vi "FTW-Actor-Core-Initialize.vi"(0 "FTW Actor Instance":refnum<class "FTW-Actor-Instance.lvclass">, 5 "Inbox Configuration":string, 7 "Primary Inbox Address":string, 9 "Actor Identity":string, 11 "error in":errorcluster) -> (4 "FTW Actor Instance out":refnum<class "FTW-Actor-Instance.lvclass">, 6 "Incoming Request":refnum<event-registration>, 8 "Resolved Primary Inbox Address":string, 15 "error out":errorcluster)   [LabVIEW 2015, in "FTW-Actor-Instance.lvclass"]
uses:
  FTW-Actor-Instance.lvclass
  core/type/FTW-Type-JSON.ctl
panel:
  # "Inputs"
  # "Outputs"
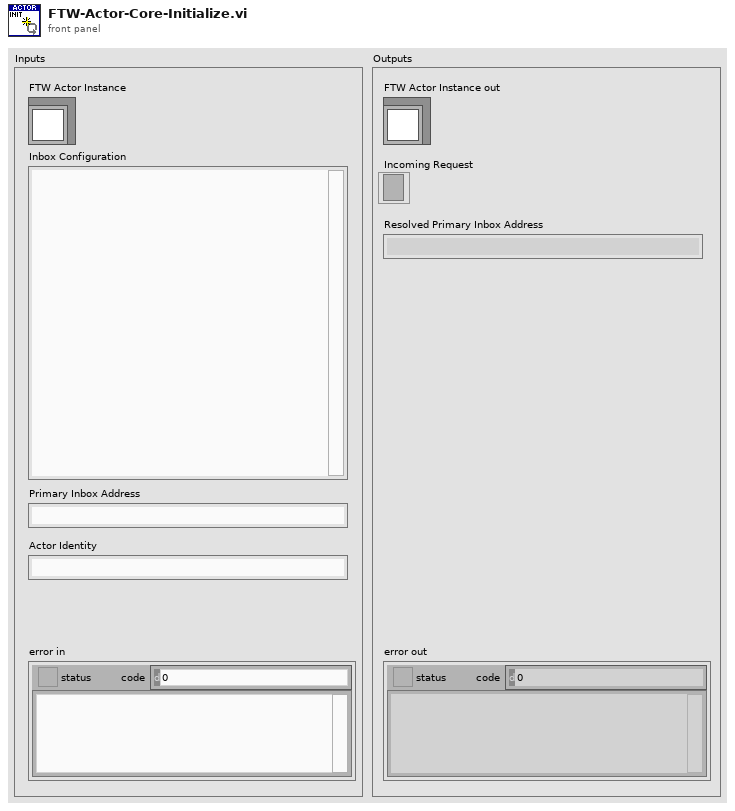
[diagram p1: front panel]
types:
  T1 = typedef "FTW-Type-JSON.ctl" = refnum<data-value>
  T2 = typedef "FTW-Type-Actor-Inbox.ctl" = refnum<data-value>
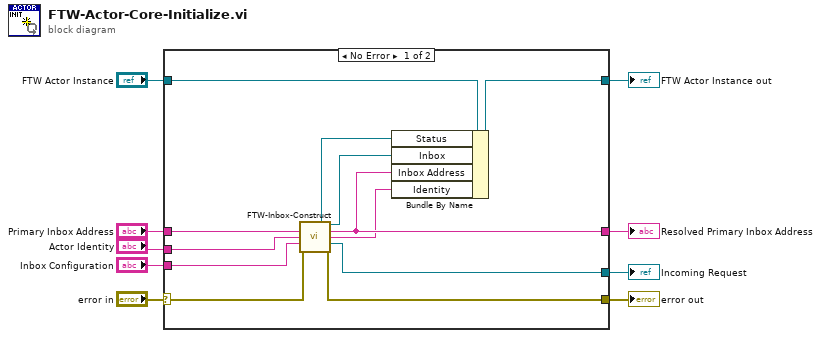
[diagram p0: block diagram]
diagram:
  n1 = case shown="No Error" "error in" {
    selector: "error in" -> [w18 w22]
    tunnel: "FTW Actor Instance" -> [w21 w23]
    tunnel: [w14 _] -> w8
    tunnel: [w20 w23] -> w7
    tunnel: [w10 w22] -> w5
    tunnel: "Inbox Configuration" -> [w13 _]
    tunnel: [w16 _] -> w3
    tunnel: "Primary Inbox Address" -> [w17 _]
    tunnel: "Actor Identity" -> [w11 _]
    frame No Error {
      n2 = call "FTW-Inbox-Construct.vi"("Primary Inbox Address"=w17, "Actor Identity"=w11, "Inbox Configuration"=w13, "error in"=w18) -> ("ActorStatus"=w15:T1, "FTW Actor Inbox"=w19:T2, "Resolved Primary Inbox Address"=w16:string, "Resolved Actor Identity"=w12:string, "Incoming Request"=w14:refnum<event-registration>, "error out"=w10:errorcluster)  [unwired: 6 in]
      n3 = Bundle By Name(cluster=w21, "Status"=w15, "Inbox"=w19, "Inbox Address"=w16, "Identity"=w12) -> (w20:refnum<class "FTW-Actor-Instance.lvclass">)
    }
    frame Error {
    }
  }
  "FTW Actor Instance out" <- w7
  "error out" <- w5
  "Incoming Request" <- w8
  "Resolved Primary Inbox Address" <- w3
